vi "SCE_parse_VIC_registry.vi"(11 "$D000 - $D03F":u8[](array[numeric]) format="%.0x") -> (3 "VIC-II":T1)   [LabVIEW 2018]
uses:
  SCE_VIC-II_registry.ctl
panel:
  # "11"
  # "16"
  # "18"
  # "20"
  # "21"
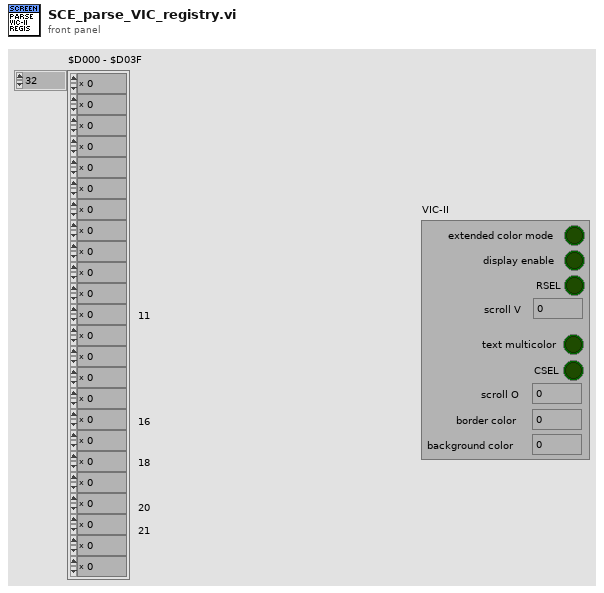
[diagram p1: front panel]
types:
  T1 = typedef "SCE_VIC-II_registry.ctl" = cluster{"extended color mode":bool, "display enable":bool, "RSEL":bool, "scroll V":u8, "text multicolor":bool, "CSEL":bool, "scroll O":u8, "border color":u8, "background color":u8}
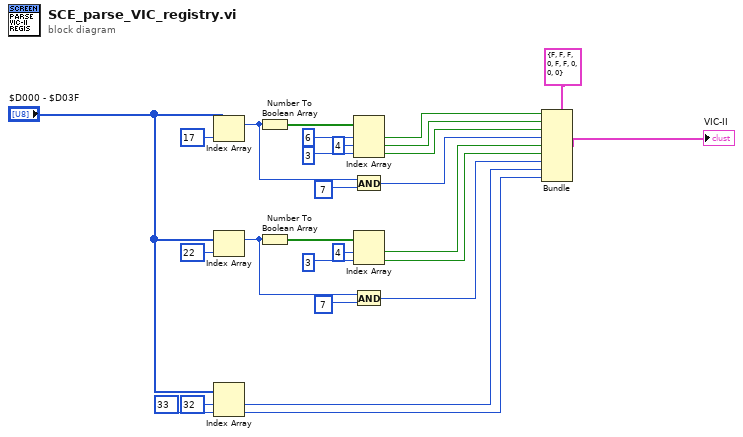
[diagram p0: block diagram]
diagram:
  n1 = Index Array(array="$D000 - $D03F", index=17) -> (element=w17:u8)
  n2 = Index Array(array="$D000 - $D03F", index=22) -> (element=w13:u8)
  n3 = Index Array(array="$D000 - $D03F", index #1=32 ("index"), index #2=33 ("index")) -> (element #1=w2:u8, element #2=w1:u8)
  n4 = Number To Boolean Array(number=w17) -> (Boolean array=w24:bool[])
  n5 = Number To Boolean Array(number=w13) -> (Boolean array=w10:bool[])
  n6 = Index Array(array=w24, index #1=6 ("index"), index #2=4 ("index"), index #3=3 ("index")) -> (element #1=w22:bool, element #2=w20:bool, element #3=w18:bool)
  n7 = And(x=w17, y=u8 7 ("index")) -> (x .and. y?=w15:u8)
  n8 = Index Array(array=w10, index #1=4 ("index"), index #2=3 ("index")) -> (element #1=w8:bool, element #2=w7:bool)
  n9 = And(x=w13, y=u8 7 ("index")) -> (x .and. y?=w6:u8)
  n10 = Bundle(cluster=T1 {"extended color mode"=FALSE, "display enable"=FALSE, "RSEL"=FALSE, "scroll V"=0, "text multicolor"=FALSE, "CSEL"=FALSE, "scroll O"=0, "border color"=0, "background color"=0} ("VIC-II"), "extended color mode"=w22, "display enable"=w20, "RSEL"=w18, "scroll V"=w15, "text multicolor"=w8, "CSEL"=w7, "scroll O"=w6, "border color"=w2, "background color"=w1) -> (→"VIC-II":T1)
